vi "AWAC_Decoder.vi"() -> ()   [LabVIEW 2016]
panel:
  out "resulting string":string
  out "Array":string[](array[string])
  out "Decoded Values":dbl[](array[numeric])
  out "Station ID":string
  in  "EXIT":bool
  in  "DECODE":bool
  out "Decoded Message":string="01 05 2017 17 32 00 00000000 01110000  14.8    0.0 155.6   3.8  -1.0   0.012  19.50     0     0\n  -3.030  -1.720   2.100  22.0  25.0  19.0\n  -4.000  -3.850   2.160  21.0  24.0  19.0\n  -4.090  -3.570   1.830  21.0  24.0  19.0\n  -3.910  -3.530   2.120  21.0  24.0  19.0\n  -3.730  -4.150   2.110  21.0  24.0  19.0"
  in  "GOES Message":string="CA99999321-@A@E_a@Q@B@@@@@_??BT@@@X_@f?v@O^M@@@@@@+?KV?jp@^@@V@Y@T+?@P?Rv@_P@U@X@S+~?r?S|@^^@U@X@S+~yv?JZ@bb@U@X@S+~?r?QR@aH@U@X@S"
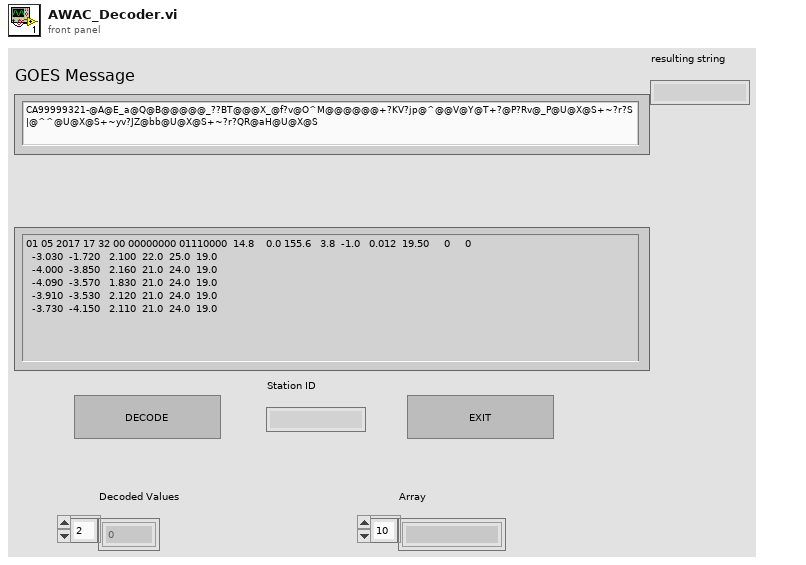
[diagram p1: front panel]
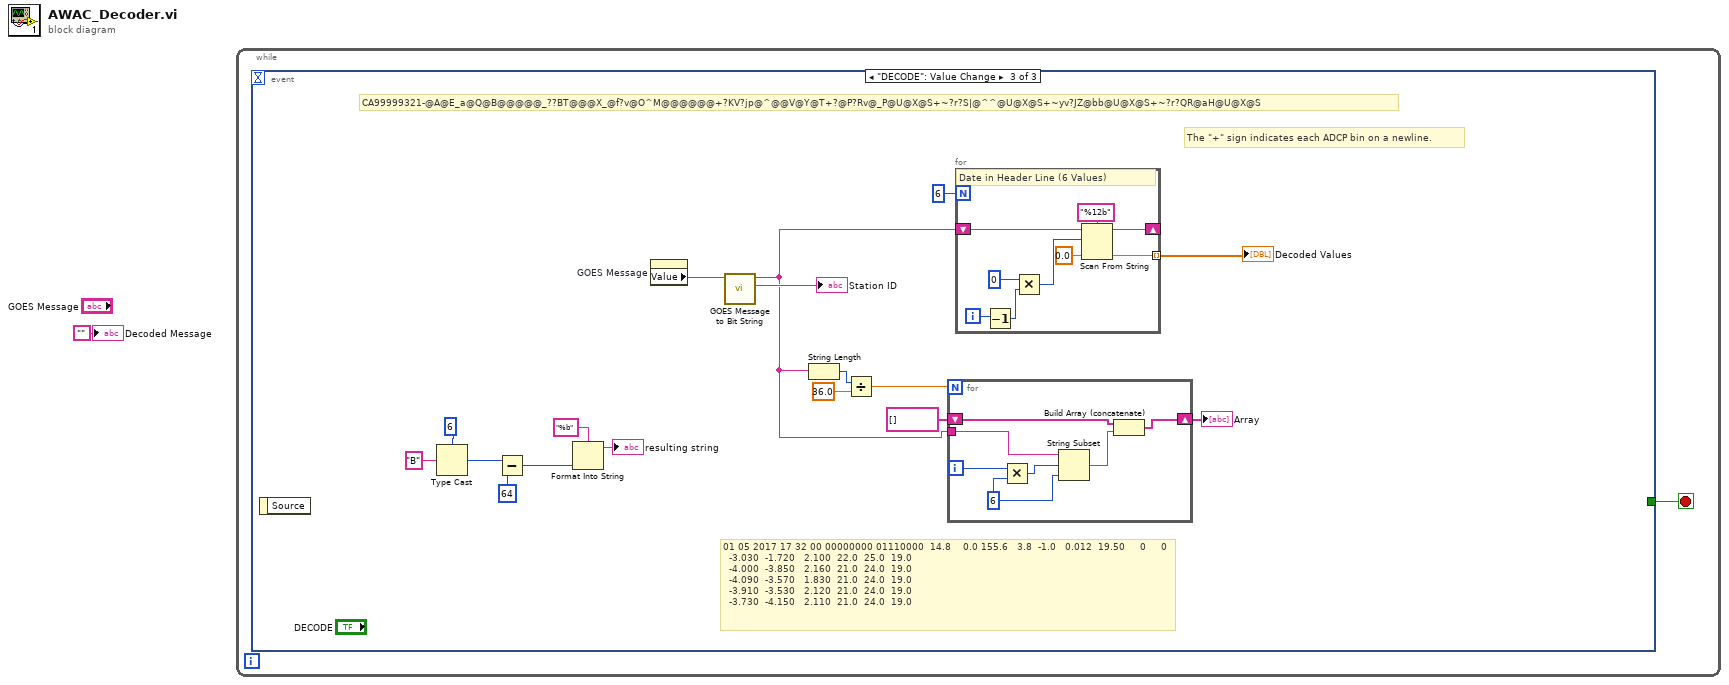
[diagram p0: block diagram]
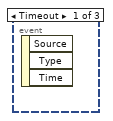
[diagram p2: hidden frame]
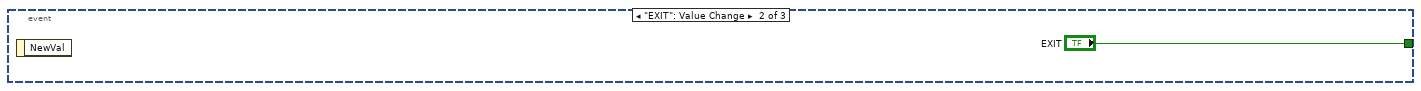
[diagram p3: hidden frame]
diagram:
  n1 = while {
    stop <- w2 stop-if-true
    n2 = event shown="[2] \"DECODE\": Value Change" {
      selector: _ -> [_ _ _]
      dyn-events: _ -> [_ _ _]
      timeout: _ -> [_ _ _]
      tunnel: [_ "EXIT" _] -> w2
      event Timeout {
        n3 = event-data() -> ()  [unwired: 1 in, 3 out]
      }
      event "EXIT": Value Change {
        n4 = event-data() -> ()  [unwired: 1 in, 1 out]
      }
      event "DECODE": Value Change {
        # "The \"+\" sign indicates each ADCP bin on a newline."
        # "CA99999321-@A@E_a@Q@B@@@@@_??BT@@@X_@f?v@O^M@@@@@@+?KV?jp@^@@V@Y@T+?@P?Rv@_P@U@X@S+~?r?S|@^^@U@X@S+~yv?JZ@bb@U@X@S+~?r?QR@aH@U@X@S"
        # "01 05 2017 17 32 00 00000000 01110000  14.8    0.0 155.6   3.8  -1.0   0.012  19.50     0     0\n  -3.030  -1.720   2.100  22.0  25.0  19.0\n  -4.000  -3.850   2.160  21.0  24.0  19.0\n  -4.090  -3.570   1.830  21.0  24.0  19.0\n  -3.910  -3.530   2.120  21.0  24.0  19.0\n  -3.730  -4.150   2.110  21.0  24.0  19.0"
        n5 = event-data() -> ()  [unwired: 1 in, 1 out]
        n6 = Type Cast(type=u8 6 ("length (rest)"), x="B") -> (*(type *) &x=w11:u8)
        n7 = Subtract(x=w11, y=u8 64 ("length (rest)")) -> (x-y=w8:u8)
        n8 = Format Into String(format string="%b", w8) -> (resulting string=→"resulting string":string)  [unwired: 2 in, 1 out]
        n9 = property on="GOES Message" class="Str"() -> ("Value"=w20:string)  [unwired: 2 in, 2 out]
        n10 = call "GOES Message to Bit String.vi"("GOES Message IN"=w20) -> ("Station ID"=→"Station ID":string, "Decoded Bit String"=w5:string)  [unwired: 8 in, 1 out]
        n11 = String Length(string=w5) -> (length=w17:i32)
        n12 = Divide(x=w17, y=36.0) -> (x/y=w16:dbl)
        n13 = for {
          N: w16 -> [_]
          tunnel: w5 -> [w34]
          shift-right: [w35] -> w14
          shift-left: string[] [] -> [w36]
          i -> [w30]
          w31 = 6 ("length (rest)")
          n14 = Multiply(x=w30, y=w31) -> (x*y=w33:i32)
          n15 = String Subset(string=w34, offset (0)=w33, length (rest)=w31) -> (substring=w32:string)
          n16 = Build Array (concatenate)(w36, w32) -> (w35:string[])
        }
        "Array" <- w14
        n17 = for {
          N: 6 -> [_]
          shift-right: [w28] -> _
          shift-left: w5 -> [w22]
          tunnel: [w21] -> w6 mode=indexing
          i -> [w26]
          # "Date in Header Line (6 Values)"
          n18 = Decrement(x=w26) -> (x-1=w25:i32)
          n19 = Multiply(x=0, y=w25) -> (x*y=w24:i32)
          n20 = Scan From String(format string="%12b", input string=w22, initial scan location=w24, default 1=0.0 ("default value 1")) -> (remaining string=w28:string, output 1=w21:dbl)  [unwired: 1 in, 2 out]
        }
        "Decoded Values" <- w6
      }
    }
  }
  "Decoded Message" <- ""
